vi "Command Turn to Heading.vi"(7 "Startup":bool, 9 "Timeout":dbl=15.0, 11 "Heading":dbl=-90.0) -> (2 "Right Wheel Velocity":dbl=680.96, 3 "Left Wheel Velocity":dbl=-680.96, 4 "Reint":bool, 6 "Completed":bool)   [LabVIEW 2017]
uses:
  Command Execution State.ctl
  Utility VIs/Refnum Names.vi
  <vilib>/Rock Robotics/WPI/ThirdParty/Phoenix-LabVIEW/Pigeon IMU/CTRE_PigeonIMU_GetRawGyro.vi
  Drive/Drive Globals.vi
  Autonomous Globals.vi
panel:
  out "Using Lower?":bool=TRUE
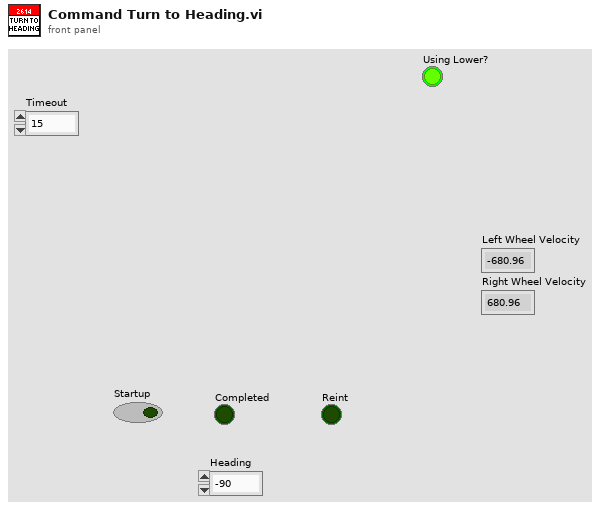
[diagram p1: front panel]
types:
  T1 = typedef "Command Execution State.ctl" = enum16{"Initialize", "Execute", "Finish"}
  T2 = typedef "CTRE_PigeonIMU_DeviceRef.ctl" = cluster{"DeviceStatus":errorcluster, "Device Number":u8, "Type":T3, "Device ID":u32, "Handle":u64, "UsageFrame":u32, "Library Path":path}
  T3 = typedef "CTRE_PigeonIMU_ConnectionType.ctl" = u32
  T4 = cluster{"X":dbl, "Y":dbl, "Z":dbl, "Magnitude":dbl}
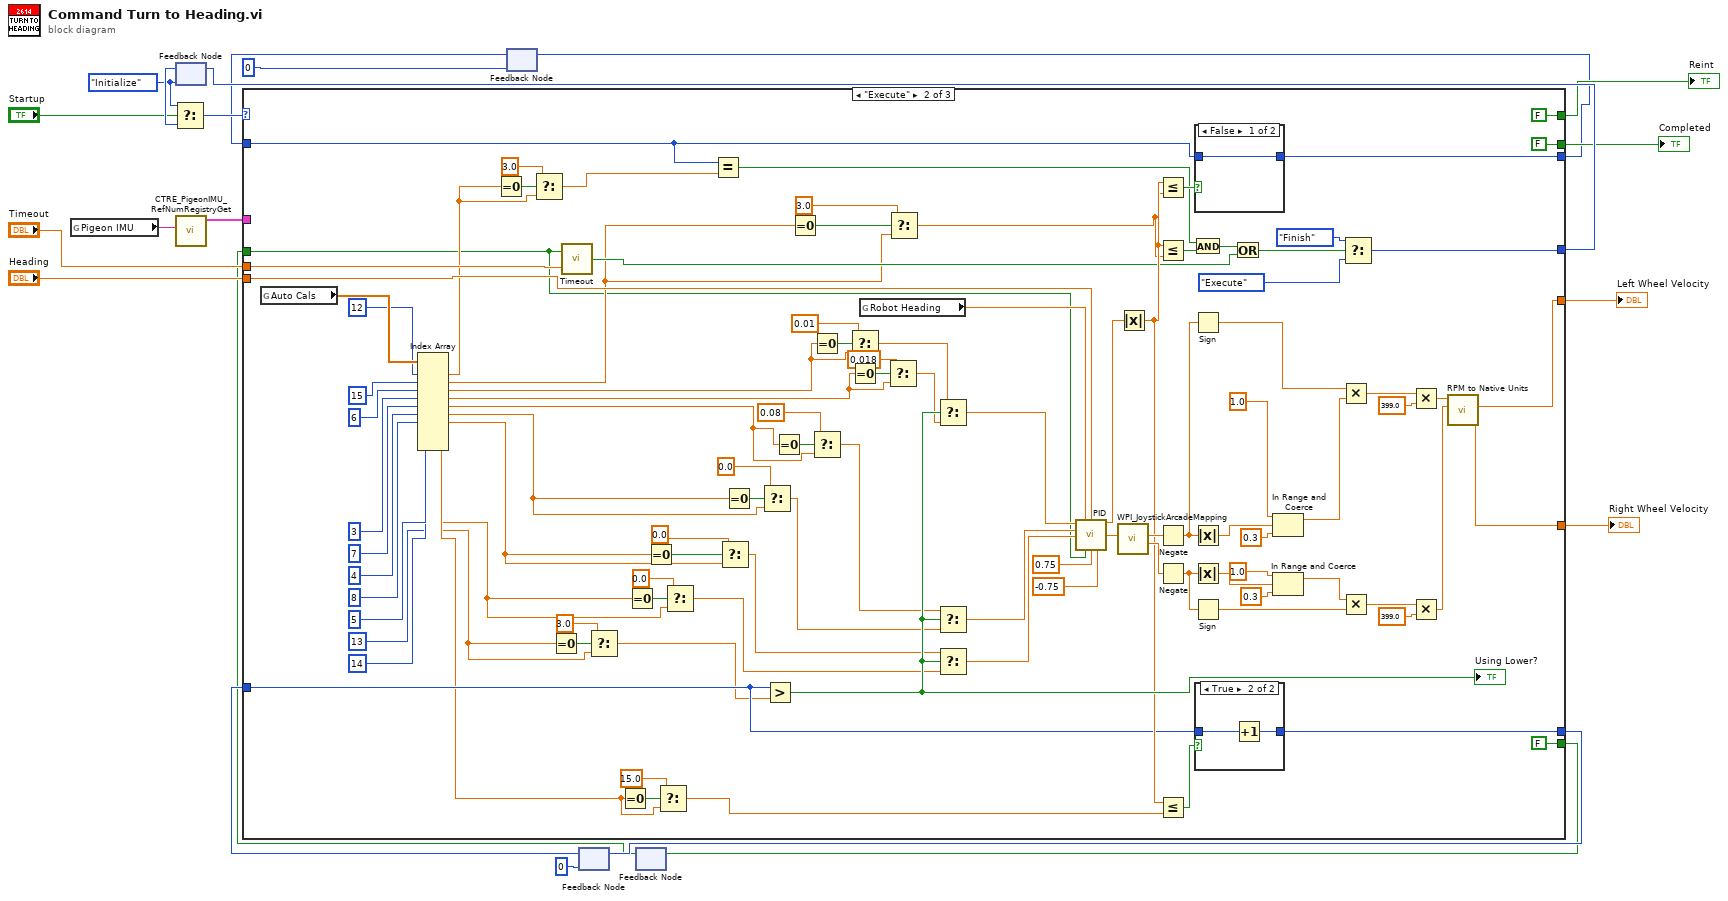
[diagram p0: block diagram]
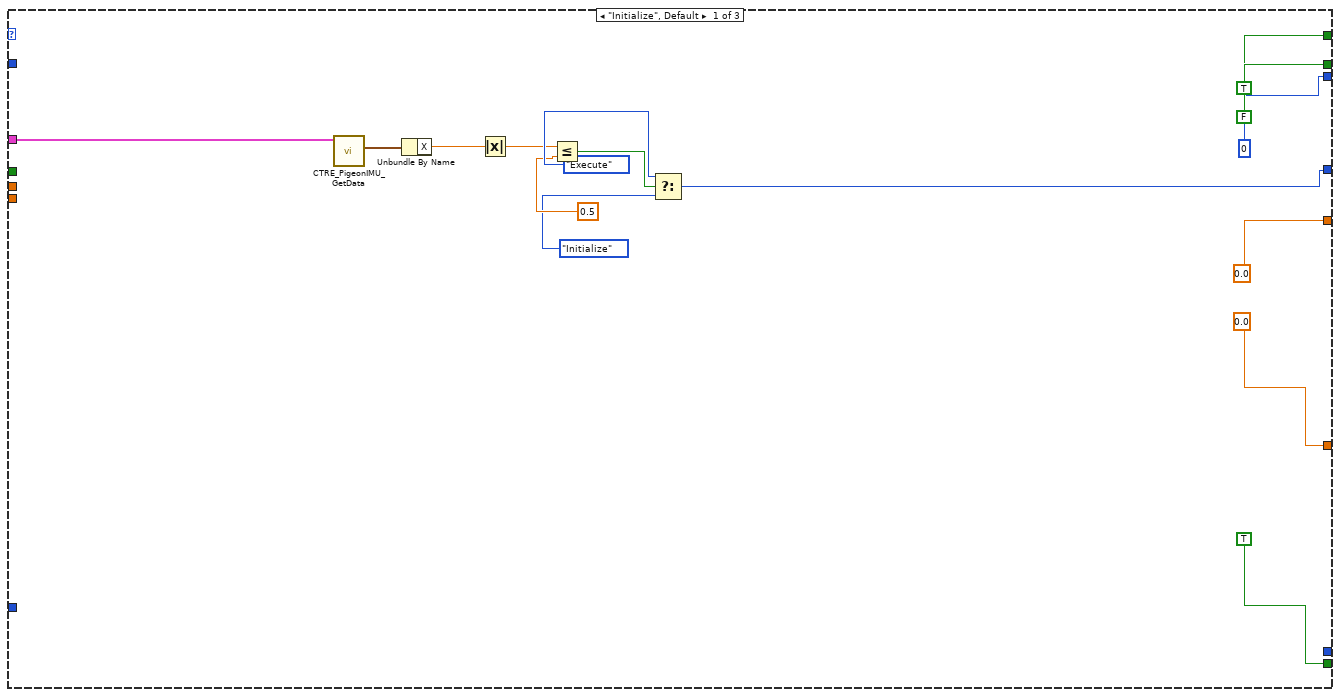
[diagram p2: hidden frame]
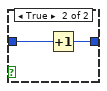
[diagram p4: hidden frame]
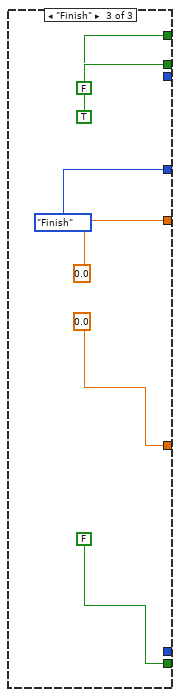
[diagram p5: hidden frame]
diagram:
  w17 = Command_Execution_State."Initialize" ("Play State")
  n1 = global read "Refnum Names.vi" "Pigeon IMU"() -> (w8:string)
  n2 = feedback #1(w17) -> (w19:T1)
  n3 = Select(t=w17, s="Startup", f=w19) -> (s? t:f=w21:T1)
  n4 = call <vilib>:"CTRE_PigeonIMU_RefNumRegistryGet.vi"("refnum name"=w8) -> ("PigeonIMUDevRef"=w7:T2)  [unwired: 9 in, 1 out]
  n5 = feedback #2(0) -> (w10:i32)
  n6 = feedback #3(0 ("y")) -> (w6:i32)
  n7 = feedback #4() -> (w1:bool)  [unwired: 1 in]
  n8 = case shown="\"Execute\"" w21 {
    tunnel: [w28 w136 Command_Execution_State."Finish" ("Play State")] -> w20
    tunnel: "Heading" -> [_ w133 _]
    tunnel: [FALSE FALSE TRUE] -> w16
    tunnel: [TRUE FALSE FALSE] -> w14
    tunnel: [0.0 w90 0.0] -> w13
    tunnel: [0.0 w89 0.0] -> w12
    tunnel: w10 -> [_ w124 _]
    tunnel: [0 w125 _] -> w9
    tunnel: w7 -> [w30 _ _]
    tunnel: w6 -> [_ w111 _]
    tunnel: [_ w112 _] -> w5
    tunnel: "Timeout" -> [_ w96 _]
    tunnel: [TRUE FALSE FALSE] -> w2
    tunnel: w1 -> [_ w37 _]
    frame "Initialize", Default {
      n9 = call-poly <vilib>:"CTRE_PigeonIMU_GetData.vi"("PigeonIMUDevRef"=w30) -> ("Gyro DPS"=w31:T4)  [unwired: 8 in, 2 out]
      n10 = Unbundle By Name(w31) -> ("X"=w27:dbl)
      n11 = Absolute Value(x=w27) -> (abs(x)=w25:dbl)
      n12 = Less Or Equal?(x=w25, y=0.5) -> (x <= y?=w24:bool)
      n13 = Select(t=Command_Execution_State."Execute" ("Play State"), s=w24, f=Command_Execution_State."Initialize") -> (s? t:f=w28:T1)
    }
    frame "Execute" {
      n14 = global read "Autonomous Globals.vi" "Auto Cals"() -> (w88:dbl[])
      n15 = Index Array(array=w88, index #1=12 ("index"), index #2=15 ("index"), index #3=6 ("index"), index #4=3 ("index"), index #5=7 ("index"), index #6=4 ("index"), index #7=8 ("index"), index #8=5 ("index"), index #9=13 ("index"), index #10=14 ("index")) -> (element #1=w75:dbl, element #2=w70:dbl, element #3=w43:dbl, element #4=w40:dbl, element #5=w47:dbl, element #6=w52:dbl, element #7=w55:dbl, element #8=w59:dbl, element #9=w62:dbl, element #10=w66:dbl)
      n16 = Equal To 0?(x=w75) -> (x = 0?=w76:bool)
      n17 = Select(t=3.0, s=w76, f=w75) -> (s? t:f=w77:dbl)
      n18 = Equal To 0?(x=w62) -> (x = 0?=w65:bool)
      n19 = call "Timeout.vi"("Timeout"=w96, "Initialize"=w37) -> ("Timed Out?"=w94:bool)
      n20 = Select(t=3.0, s=w65, f=w62) -> (s? t:f=w63:dbl)
      n21 = Equal To 0?(x=w66) -> (x = 0?=w69:bool)
      n22 = Equal To 0?(x=w59) -> (x = 0?=w60:bool)
      n23 = Equal To 0?(x=w55) -> (x = 0?=w57:bool)
      n24 = Select(t=15.0, s=w69, f=w66) -> (s? t:f=w67:dbl)
      n25 = Select(t=0.0, s=w60, f=w59) -> (s? t:f=w58:dbl)
      n26 = Equal?(x=w124, y=w77) -> (x = y?=w117:bool)
      n27 = Select(t=0.0, s=w57, f=w55) -> (s? t:f=w54:dbl)
      n28 = Equal To 0?(x=w52) -> (x = 0?=w51:bool)
      n29 = Select(t=0.0, s=w51, f=w52) -> (s? t:f=w50:dbl)
      n30 = Greater?(x=w111, y=w63) -> (0:w118:bool)
      "Using Lower?" <- w118
      n31 = Equal To 0?(x=w47) -> (x = 0?=w49:bool)
      n32 = Equal To 0?(x=w70) -> (x = 0?=w73:bool)
      n33 = Equal To 0?(x=w43) -> (x = 0?=w44:bool)
      n34 = Select(t=0.08, s=w49, f=w47) -> (s? t:f=w46:dbl)
      n35 = Select(t=0.01, s=w44, f=w43) -> (s? t:f=w41:dbl)
      n36 = Equal To 0?(x=w40) -> (x = 0?=w42:bool)
      n37 = global read "Drive Globals.vi" "Robot Heading"() -> (w132:dbl)
      n38 = Select(t=0.018, s=w42, f=w40) -> (s? t:f=w38:dbl)
      n39 = Select(t=3.0, s=w73, f=w70) -> (s? t:f=w71:dbl)
      n40 = Select(t=w41, s=w118, f=w38) -> (s? t:f=w121:dbl)
      n41 = Select(t=w46, s=w118, f=w50) -> (s? t:f=w119:dbl)
      n42 = Select(t=w54, s=w118, f=w58) -> (s? t:f=w120:dbl)
      n43 = call "PID.vi"("Kp"=w121, "Process Variable"=w132, "Goal"=w133, "Ki"=w119, "Kd"=w120, "Reinit"=w37, "Max Ouput"=0.75, "Min Output"=-0.75) -> ("Current Error"=w134:dbl, "Command"=w130:dbl)  [unwired: 5 in, 1 out]
      n44 = call <vilib>:"WPI_JoystickArcadeMapping.vi"("X axis value"=w130) -> ("Right Motor Value"=w128:dbl, "Left Motor Value"=w129:dbl)  [unwired: 9 in]
      n45 = Absolute Value(x=w134) -> (abs(x)=w114:dbl)
      n46 = Less Or Equal?(x=w114, y=w71) -> (x <= y?=w131:bool)
      n47 = Less Or Equal?(x=w114, y=w71) -> (x <= y?=w115:bool)
      n48 = Negate(x=w129) -> (-x=w100:dbl)
      n49 = Negate(x=w128) -> (-x=w99:dbl)
      n50 = Less Or Equal?(x=w114, y=w67) -> (x <= y?=w113:bool)
      n51 = And(x=w117, y=w115) -> (x .and. y?=w116:bool)
      n52 = Sign(1:w100) -> (0:w108:dbl)
      n53 = Absolute Value(x=w100) -> (abs(x)=w110:dbl)
      n54 = Absolute Value(x=w99) -> (abs(x)=w109:dbl)
      n55 = Sign(1:w99) -> (0:w105:dbl)
      n56 = case shown="False" w131 {
        tunnel: w124 -> [w143 w145]
        tunnel: [w143 w144] -> w125
        frame False {
        }
        frame True {
          n57 = Increment(x=w145) -> (x+1=w144:i32)
        }
      }
      n58 = case shown="True" w113 {
        tunnel: w111 -> [w140 w142]
        tunnel: [w140 w141] -> w112
        frame False {
        }
        frame True {
          n59 = Increment(x=w142) -> (x+1=w141:i32)
        }
      }
      n60 = Or(x=w116, y=w94) -> (x .or. y?=w95:bool)
      n61 = In Range and Coerce(upper limit=1.0, x=w110, lower limit=0.3) -> (coerced(x)=w107:dbl)  [unwired: 1 out]
      n62 = In Range and Coerce(upper limit=1.0, x=w109, lower limit=0.3) -> (coerced(x)=w106:dbl)  [unwired: 1 out]
      n63 = Multiply(x=w108, y=w107) -> (x*y=w97:dbl)
      n64 = Multiply(x=w106, y=w105) -> (x*y=w98:dbl)
      n65 = Select(t=Command_Execution_State."Finish" ("Play State"), s=w95, f=Command_Execution_State."Execute") -> (s? t:f=w136:T1)
      n66 = Multiply(x=w97, y=399.0) -> (x*y=w92:dbl)
      n67 = Multiply(x=w98, y=399.0) -> (x*y=w91:dbl)
      n68 = call "RPM to Native Units.vi"("Right RPM"=w91, "Left RPM"=w92) -> ("Right Out"=w89:dbl, "Left Out"=w90:dbl)  [unwired: 6 in, 1 out]
    }
    frame "Finish" {
    }
  }
  "Completed" <- w16
  "Reint" <- w14
  "Left Wheel Velocity" <- w13
  "Right Wheel Velocity" <- w12
  n69 = feedback-in #1(w20) -> ()
  n70 = feedback-in #2(w9) -> ()
  n71 = feedback-in #3(w5) -> ()
  n72 = feedback-in #4(w2) -> ()
